vi "DFD FXP MRate Quantization.vi"(5 "scale by power of 2? (F)":bool, 6 "gain settings":T1={"gain processing"=1, "gain word length"=16} {"gain processing" items=["On Target", "On Host"]}, 7 "scale type":T2=enum."Time Domain 1-Norm", 8 "error in (no error)":errorcluster, 10 "coefficients word length":i16=16, 11 "multirate filter in":T3={"mMRate_Structure"=enum."IIR", "mMRate_Mode"=0, "mMRate_Factor"=-1, "mMRate_FIRParams"={"mMRate_FIR_H"=[], "mMRate_FIR_IsNyquist?"=FALSE, "mMRate_FIR_IsSymmetric?"=FALSE}, "mMRate_CICParams"={"mMRate_CIC_#Stage"=0, "mMRate_CIC_Lag"=0, "mMRate_CIC_Type"=enum."Lowpass"}, "mMRate_Order"=0, "mMRate_Version"="2.0", "mMRate_Comments"="", "mMRate_RationalFactor"={"mMRate_L"=-1, "mMRate_M"=-1}, "mMRate_Fs"=1.0, "mMRate_Quantized?"=FALSE, "mMRate_QFilterGain"=1.0, "mMRate_CoefWl"=16, "mMRate_Scaling"={"mMRate_ScaleByPowerOf2?"=FALSE, "mMRate_ScaleType"=enum."No Norm"}, "mMRate_InputWl"=16, "mMRate_OutputWl"=16, "mMRate_OutputMode"=enum."Truncation", "mMRate_MultMode"=enum."Truncated", "mMRate_BitPruning"=FALSE, "mMRate_GainWl"=16, "mMRate_OutputFwl"=0, "mMRate_SumIwl"=0, "mMRate_InputIwl "=16, "mMRate_SumWl"=32, "mMRate_CoefIwl"=0} {"mMRate_SumWl" min=1 max=32 step=1; "mMRate_InputIwl" min=1 max=32 step=1; "mMRate_GainWl" min=1 max=32 step=1; "mMRate_OutputWl" min=1 max=32 step=1; "mMRate_InputWl" min=1 max=32 step=1; "mMRate_CoefWl" min=1 max=32 step=1; "mMRate_Mode" items=["Default"=-1, "No Rate Change"=0, "Interpolation"=1, "Decimation"=2, "Interpolated"=3, "Rational"=4]}) -> (0 "error out":errorcluster, 2 "postprocessing gain":dbl, 3 "multirate filter out":T3={"mMRate_Structure"=enum."IIR", "mMRate_Mode"=0, "mMRate_Factor"=-1, "mMRate_FIRParams"={"mMRate_FIR_H"=[], "mMRate_FIR_IsNyquist?"=FALSE, "mMRate_FIR_IsSymmetric?"=FALSE}, "mMRate_CICParams"={"mMRate_CIC_#Stage"=0, "mMRate_CIC_Lag"=0, "mMRate_CIC_Type"=enum."Lowpass"}, "mMRate_Order"=0, "mMRate_Version"="2.0", "mMRate_Comments"="", "mMRate_RationalFactor"={"mMRate_L"=-1, "mMRate_M"=-1}, "mMRate_Fs"=1.0, "mMRate_Quantized?"=FALSE, "mMRate_QFilterGain"=1.0, "mMRate_CoefWl"=16, "mMRate_Scaling"={"mMRate_ScaleByPowerOf2?"=FALSE, "mMRate_ScaleType"=enum."No Norm"}, "mMRate_InputWl"=16, "mMRate_OutputWl"=16, "mMRate_OutputMode"=enum."Truncation", "mMRate_MultMode"=enum."Truncated", "mMRate_BitPruning"=FALSE, "mMRate_GainWl"=16, "mMRate_OutputFwl"=0, "mMRate_SumIwl"=0, "mMRate_InputIwl "=16, "mMRate_SumWl"=32, "mMRate_CoefIwl"=0} {"mMRate_SumWl" min=1 max=32 step=1; "mMRate_InputIwl" min=1 max=32 step=1; "mMRate_GainWl" min=1 max=32 step=1; "mMRate_OutputWl" min=1 max=32 step=1; "mMRate_InputWl" min=1 max=32 step=1; "mMRate_CoefWl" min=1 max=32 step=1; "mMRate_Mode" items=["Default"=-1, "No Rate Change"=0, "Interpolation"=1, "Decimation"=2, "Interpolated"=3, "Rational"=4]})   [LabVIEW 2017, in "NI_DigFilterLicensed.lvlib"]
doc: "Quantizes the coefficients of a floating-point multirate filter and generates a fixed-point multirate filter."
uses:
  <vilib>/addons/Digital Filter Design/NI_DigFilterLicensed.lvlib
  <vilib>/addons/Digital Filter Design/_Objects.llb/DFD Multirate Filter Obj.ctl
  <vilib>/addons/Digital Filter Design/_Objects.llb/DFD Multirate Mode.ctl
  <vilib>/addons/Digital Filter Design/_Objects.llb/DFD Coef Norm Type.ctl
  <vilib>/addons/Digital Filter Design/_Objects.llb/DFD Round-off Mode.ctl
  <vilib>/addons/Digital Filter Design/_Objects.llb/DFD FXP MRate Multiply Mode.ctl
  <vilib>/addons/Digital Filter Design/_Objects.llb/DFD FXP MRate Internal Precision Mode.ctl
  <vilib>/addons/Digital Filter Design/_Misc.llb/dfd_Error Handlers (Single).vi
  <vilib>/addons/Digital Filter Design/NI_DigFilter_FXP.lvlib
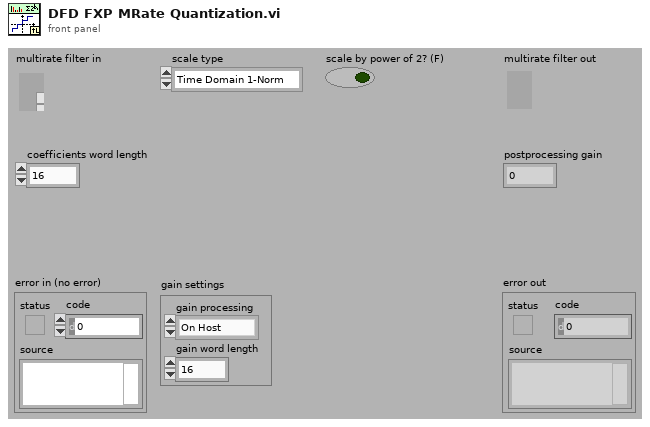
[diagram p1: front panel]
types:
  T1 = cluster{"gain processing":u16, "gain word length":i16}
  T2 = typedef "NI_DigFilterLicensed.lvlib/DFD Coef Norm Type.ctl" = enum16{"No Norm", "Time Domain 1-Norm", "Time Domain 2-Norm", "Time Domain Inf-Norm"}
  T3 = typedef "NI_DigFilterLicensed.lvlib/DFD Multirate Filter Obj.ctl" = cluster{"mMRate_Structure":enum16{"CIC", "FIR", "IIR", "Lattice"}, "mMRate_Mode":T4, "mMRate_Factor":i32, "mMRate_FIRParams":cluster{"mMRate_FIR_H":dbl[], "mMRate_FIR_IsNyquist?":bool, "mMRate_FIR_IsSymmetric?":bool}, "mMRate_CICParams":cluster{"mMRate_CIC_#Stage":i32, "mMRate_CIC_Lag":i32, "mMRate_CIC_Type":enum16{"Lowpass", "Highpass"}}, "mMRate_Order":i32, "mMRate_Version":string, "mMRate_Comments":string, "mMRate_RationalFactor":cluster{"mMRate_L":i32, "mMRate_M":i32}, "mMRate_Fs":dbl, "mMRate_Quantized?":bool, "mMRate_QFilterGain":dbl, "mMRate_CoefWl":i16, "mMRate_Scaling":cluster{"mMRate_ScaleByPowerOf2?":bool, "mMRate_ScaleType":T2}, "mMRate_InputWl":i16, "mMRate_OutputWl":i16, "mMRate_OutputMode":T5, "mMRate_MultMode":T6, "mMRate_BitPruning":bool, "mMRate_GainWl":i16, "mMRate_OutputFwl":i16, "mMRate_SumIwl":i16, "mMRate_InputIwl ":i16, "mMRate_SumWl":i16, "mMRate_CoefIwl":i16}
  T4 = typedef "NI_DigFilterLicensed.lvlib/DFD Multirate Mode.ctl" = i16
  T5 = typedef "NI_DigFilterLicensed.lvlib/DFD Round-off Mode.ctl" = enum16{"Nearest", "Truncation"}
  T6 = typedef "NI_DigFilterLicensed.lvlib/DFD FXP MRate Multiply Mode.ctl" = enum16{"Truncated", "Full"}
  T7 = typedef "NI_DigFilterLicensed.lvlib/DFD FXP MRate Internal Precision Mode.ctl" = enum16{"Truncated", "Full"}
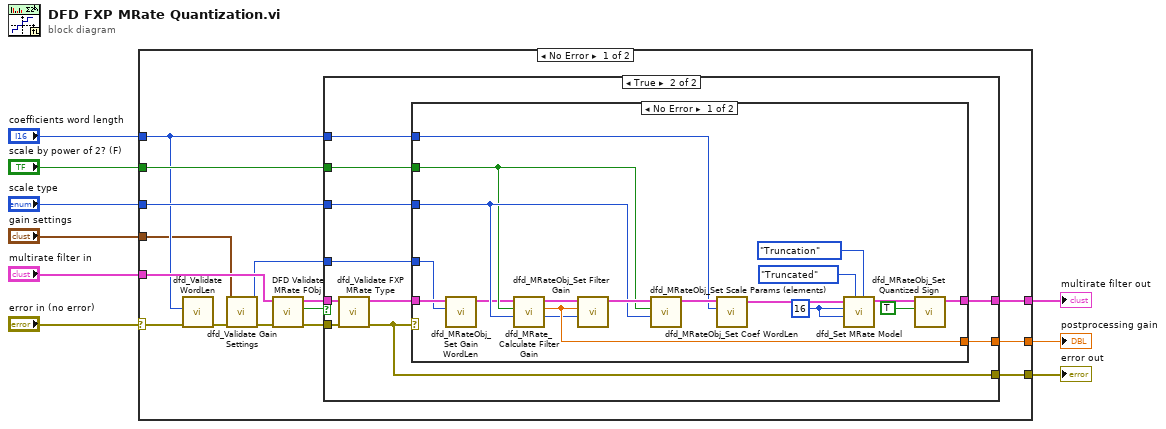
[diagram p0: block diagram]
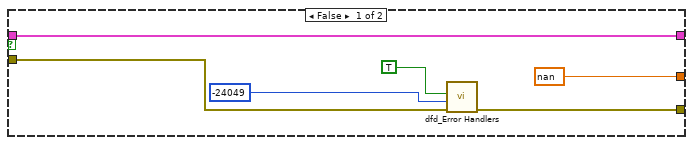
[diagram p2: hidden frame]
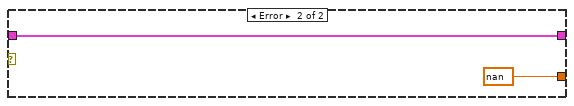
[diagram p3: hidden frame]
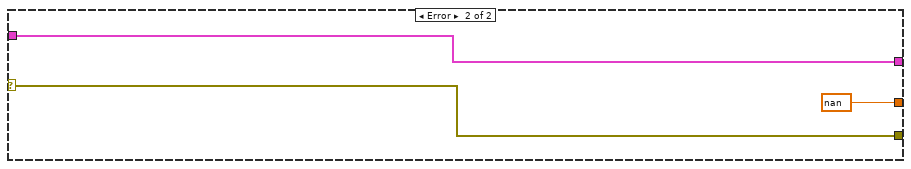
[diagram p4: hidden frame]
diagram:
  n1 = case shown="No Error" "error in (no error)" {
    selector: "error in (no error)" -> [w10 w63]
    tunnel: "multirate filter in" -> [w24 w62]
    tunnel: "scale by power of 2? (F)" -> [w20 _]
    tunnel: "scale type" -> [w19 _]
    tunnel: [w18 w62] -> w6
    tunnel: [w17 w63] -> w5
    tunnel: [w16 nan ("filter gain")] -> w4
    tunnel: "coefficients word length" -> [w15 _]
    tunnel: "gain settings" -> [w12 _]
    frame No Error {
      n2 = call <vilib>:"dfd_Validate WordLen.vi"("error in (no error)"=w10, "wl"=w15) -> ("error out"=w14:errorcluster)  [unwired: 9 out]
      n3 = call <vilib>:"dfd_Validate Gain Settings.vi"("error in (no error)"=w14, "gain setting"=w12) -> ("error out"=w13:errorcluster, "gain wl"=w11:i16)  [unwired: 8 out]
      n4 = call <vilib>:"DFD Validate MRate FObj.vi"("error in (no error)"=w13, "multirate filter in"=w24) -> ("error out"=w21:errorcluster, "is valid FLP?"=w23:bool, "multirate filter out"=w22:T3)  [unwired: 7 out]
      n5 = case shown="True" w23 {
        tunnel: w22 -> [w27 w35]
        tunnel: w21 -> [w28 w33]
        tunnel: w20 -> [_ w37]
        tunnel: w19 -> [_ w40]
        tunnel: w15 -> [_ w39]
        tunnel: [w27 w38] -> w18
        tunnel: [w26 w32] -> w17
        tunnel: [nan ("filter gain") w36] -> w16
        tunnel: w11 -> [_ w31]
        frame False {
          n6 = call-poly <vilib>:"dfd_Error Handlers.vi"("error in (no error)"=w28, "error code"=-24049 ("ERR_INVALID_MULTIRATE_FILTER"), "condition failed?"=TRUE) -> ("error out"=w26:errorcluster)  [unwired: 8 out]
        }
        frame True {
          n7 = call <vilib>:"dfd_Validate FXP MRate Type.vi"("error in (no error)"=w33, "multirate filter in"=w35) -> ("error out"=w32:errorcluster, "dup multirate filter"=w34:T3)  [unwired: 8 out]
          n8 = case shown="No Error" w32 {
            tunnel: w34 -> [w49 w59]
            tunnel: w40 -> [w56 _]
            tunnel: w39 -> [w54 _]
            tunnel: [w52 w59] -> w38
            tunnel: w37 -> [w51 _]
            tunnel: [w50 nan ("filter gain")] -> w36
            tunnel: w31 -> [w48 _]
            frame No Error {
              w45 = i16 16 ("input wl")
              n9 = call <vilib>:"dfd_MRateObj_Set Gain WordLen.vi"("gain wl"=w48, "multirate filter in"=w49) -> ("multirate filter out"=w47:T3)  [unwired: 9 out]
              n10 = call <vilib>:"dfd_MRate_Calculate Filter Gain.vi"("scale type"=w56, "scale by Power of 2?"=w51, "multirate filter in"=w47) -> ("sum iwl"=w46:i16, "scaled gain"=w50:dbl, "dup multirate filter"=w58:T3)  [unwired: 6 out]
              n11 = call <vilib>:"dfd_MRateObj_Set Filter Gain.vi"("sum iwl"=w46, "gain"=w50, "multirate filter in"=w58) -> ("multirate filter out"=w57:T3)  [unwired: 8 out]
              n12 = call <vilib>:"dfd_MRateObj_Set Scale Params (elements).vi"("scale type"=w56, "scale by Power of 2?"=w51, "multirate filter in"=w57) -> ("multirate filter out"=w55:T3)  [unwired: 8 out]
              n13 = call <vilib>:"dfd_MRateObj_Set Coef WordLen.vi"("coef wl"=w54, "multirate filter in"=w55) -> ("multirate filter out"=w41:T3)  [unwired: 9 out]
              n14 = call <vilib>:"dfd_Set MRate Model.vi"("output rounding mode"=DFD_Round-off_Mode."Truncation" ("output round-off mode"), "internal precision"=DFD_FXP_MRate_Internal_Precision_Mode."Truncated", "output wl"=w45, "input wl"=w45, "multirate filter in"=w41) -> ("multirate filter out"=w42:T3)  [unwired: 2 in, 4 out]
              n15 = call <vilib>:"dfd_MRateObj_Set Quantized Sign.vi"("Quantized?"=TRUE, "multirate filter in"=w42) -> ("multirate filter out"=w52:T3)  [unwired: 9 out]
            }
            frame Error {
            }
          }
        }
      }
    }
    frame Error {
    }
  }
  "multirate filter out" <- w6
  "error out" <- w5
  "postprocessing gain" <- w4
